vi "FaKI State Machine.vi"() -> ()   [LabVIEW 2021, in "FaKI State Machine.lvlib"]
doc: "The Producer-Consumer version of JKI State Machine.\n\nThis VI template must be instantiated by placing it on the block diagram of a new blank VI directly from the palettes. Do not use this template directly."
uses:
  FaKI State Machine.lvlib
panel:
  in  "Exit":bool
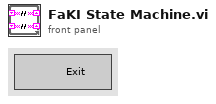
[diagram p1: front panel]
types:
  T1 = enum32{"Invalid", "Standard", "Closed", "Hidden", "Minimized", "Maximized"}
  T2 = enum32{"invalid app kind", "Development System", "Run Time System", "Student Edition", "Embedded LabVIEW", "Evaluation", "Custom"}
  T3 = cluster{"Core":cluster{"Current VI Reference":refnum<vi>, "Close Panel on Exit?":bool}, "Your Boolean data":bool, "Your string data":string}
  T4 = cluster{"Current VI Reference":refnum<vi>, "Close Panel on Exit?":bool}
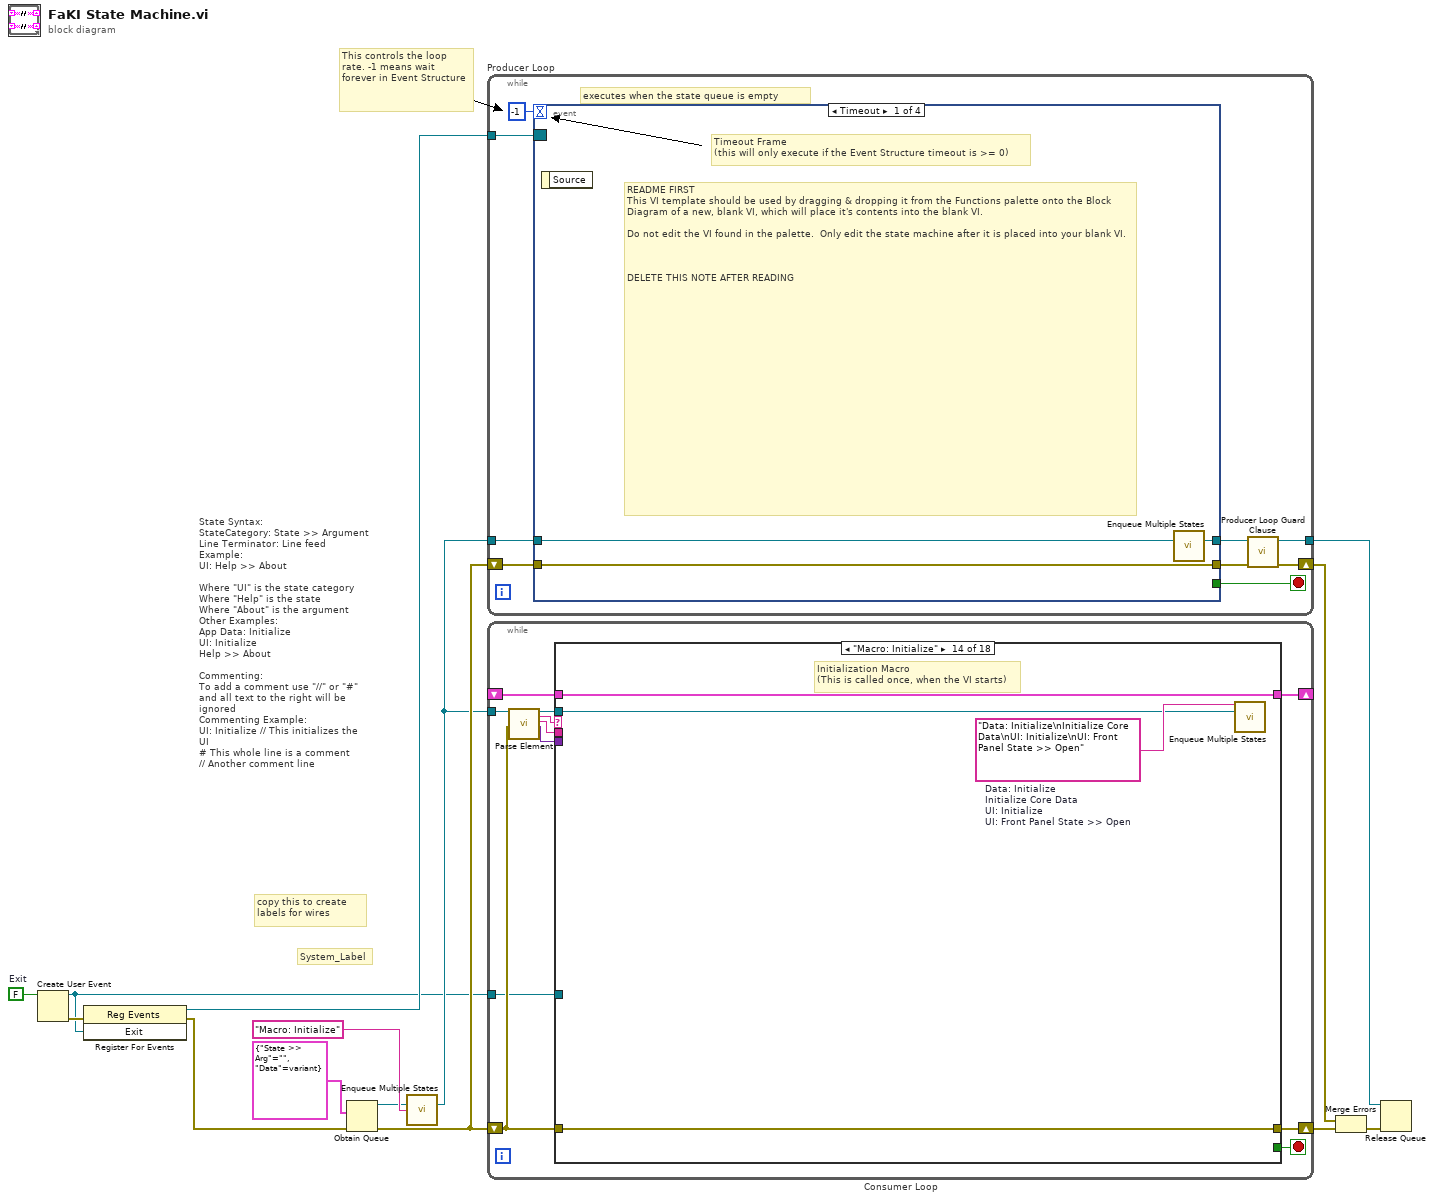
[diagram p0: block diagram]
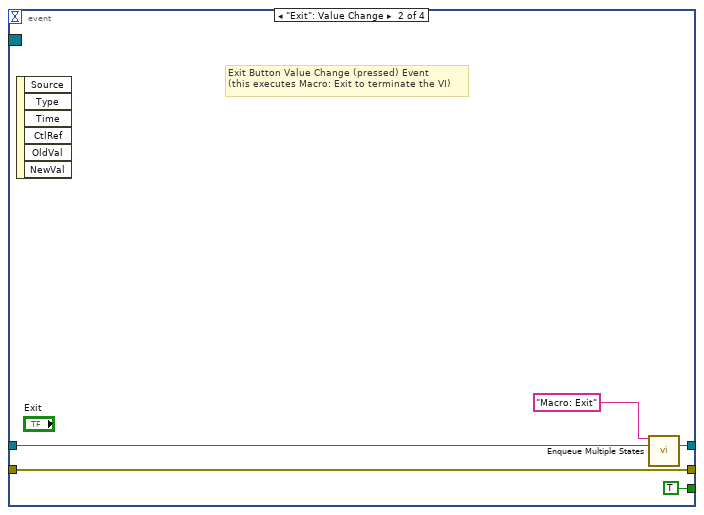
[diagram p2: hidden frame]
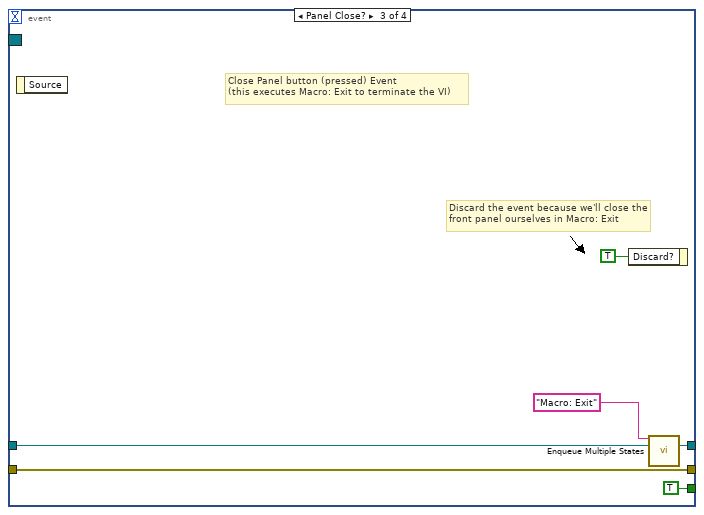
[diagram p3: hidden frame]
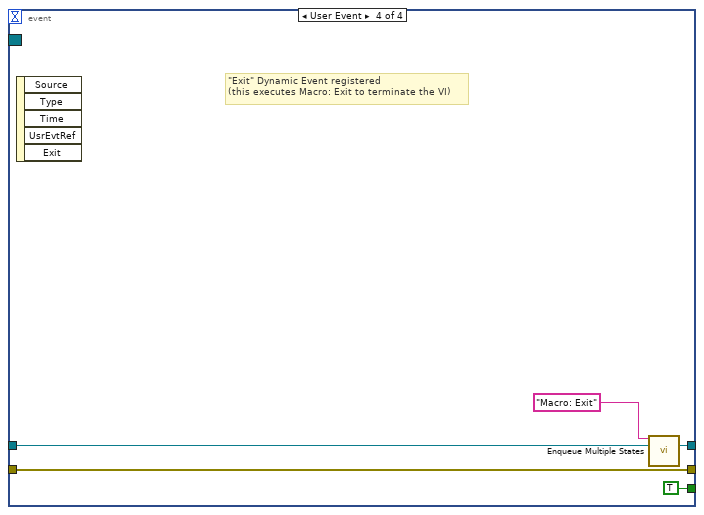
[diagram p4: hidden frame]
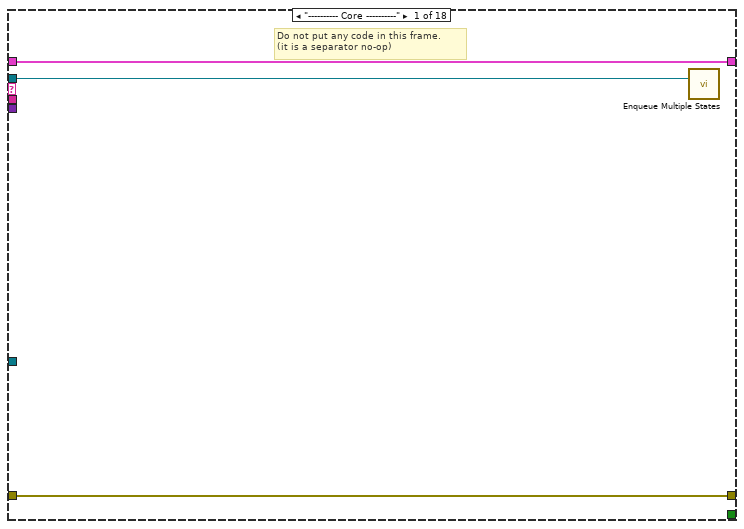
[diagram p5: hidden frame]
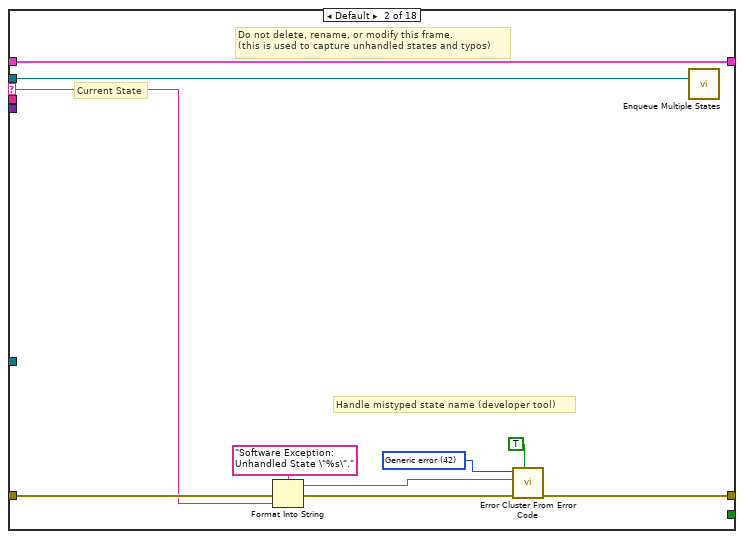
[diagram p6: hidden frame]
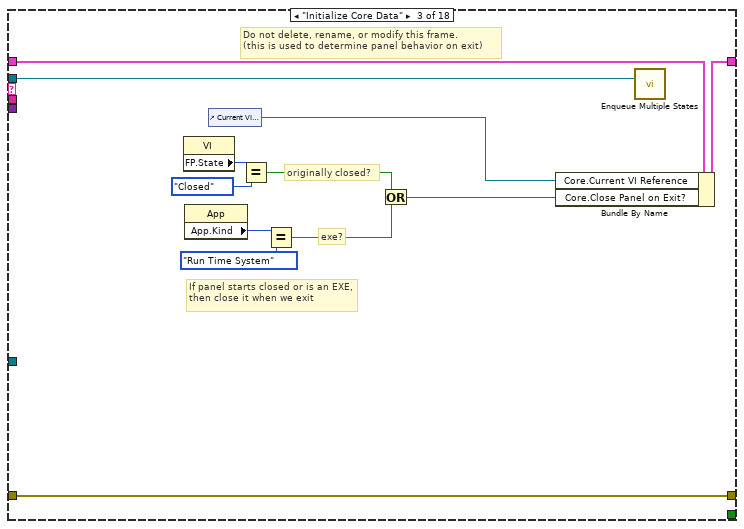
[diagram p7: hidden frame]
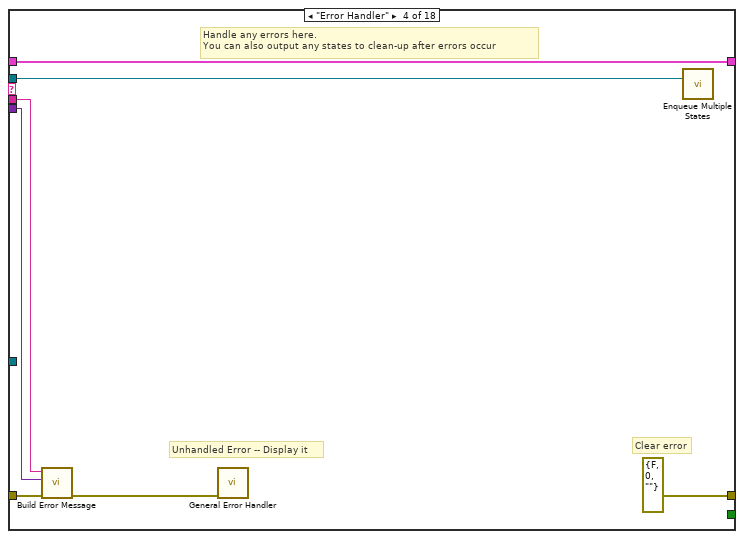
[diagram p8: hidden frame]
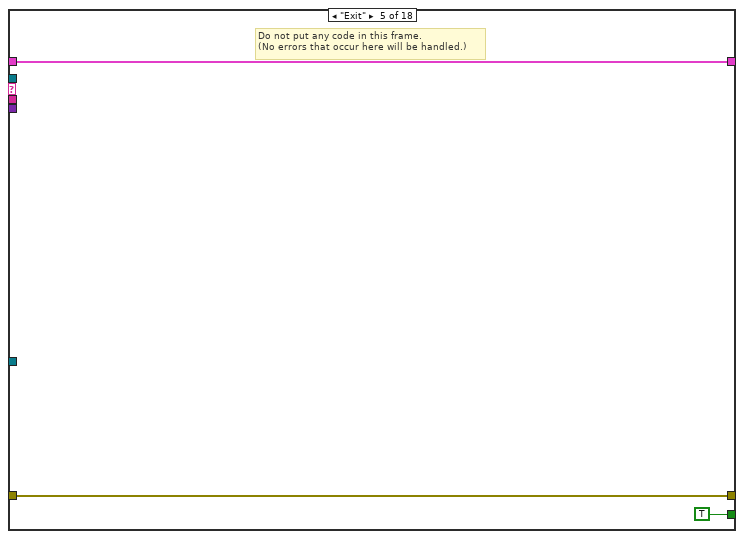
[diagram p9: hidden frame]
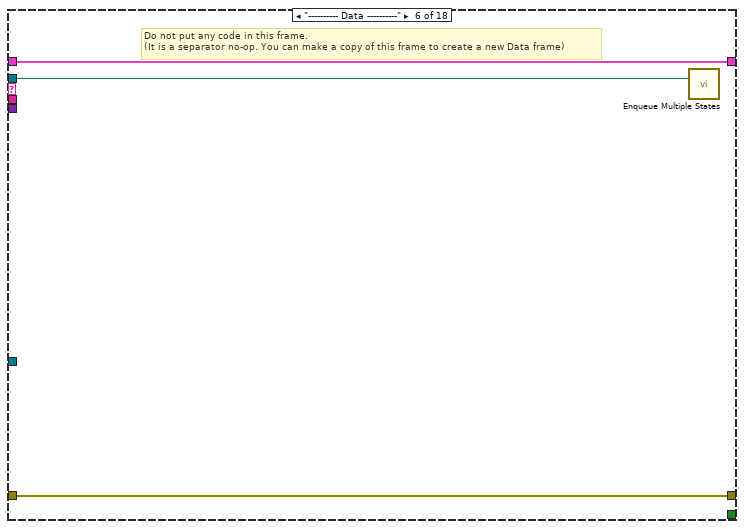
[diagram p10: hidden frame]
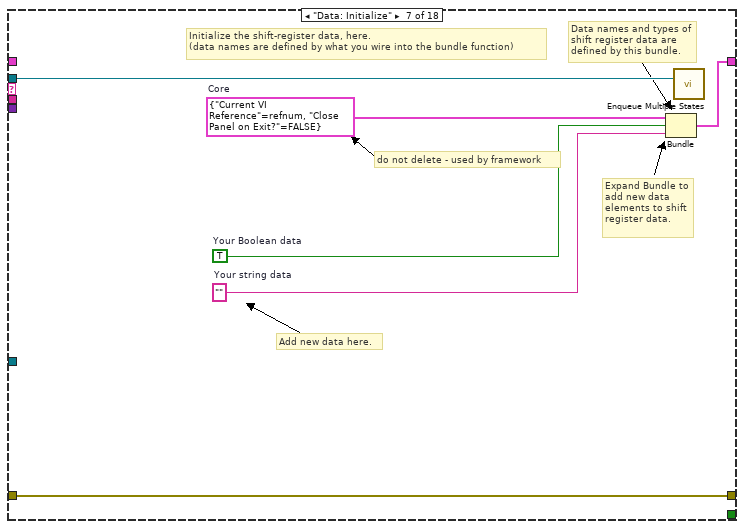
[diagram p11: hidden frame]
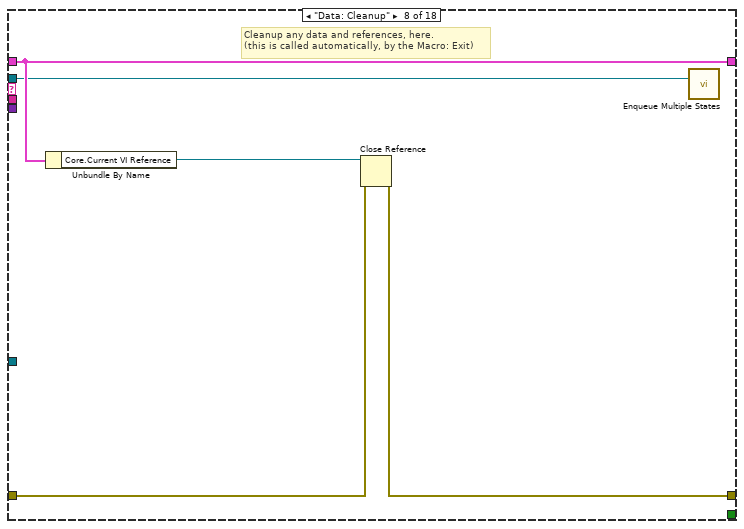
[diagram p12: hidden frame]
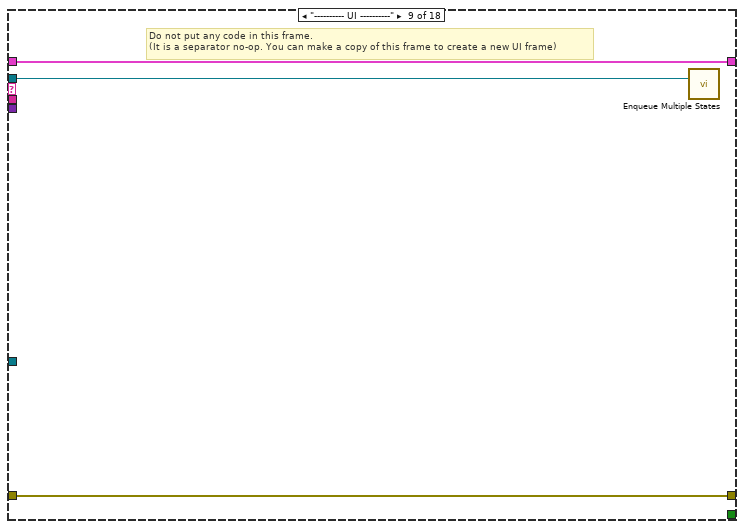
[diagram p13: hidden frame]
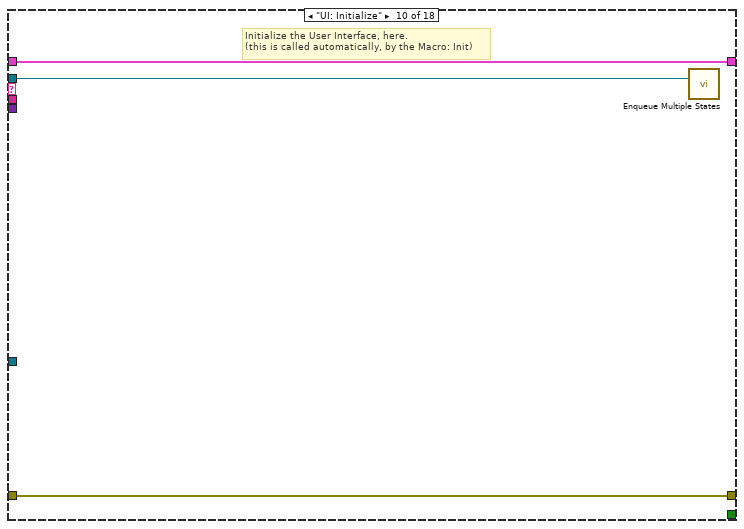
[diagram p14: hidden frame]
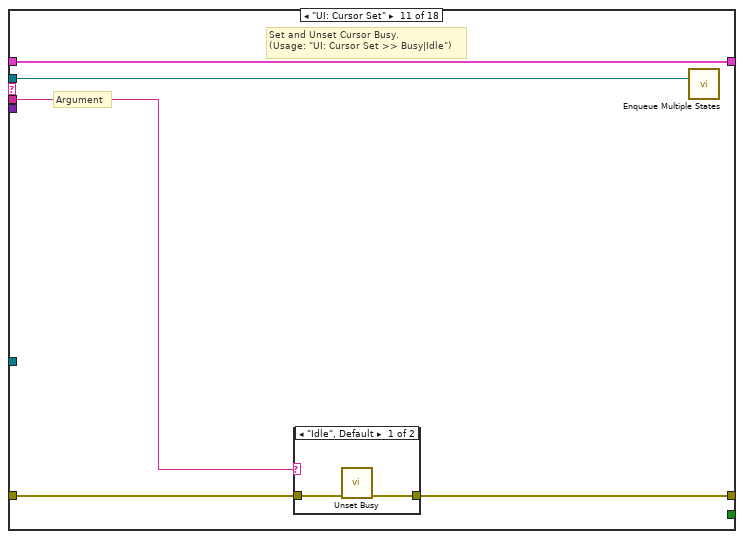
[diagram p15: hidden frame]
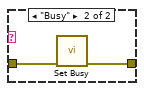
[diagram p16: hidden frame]
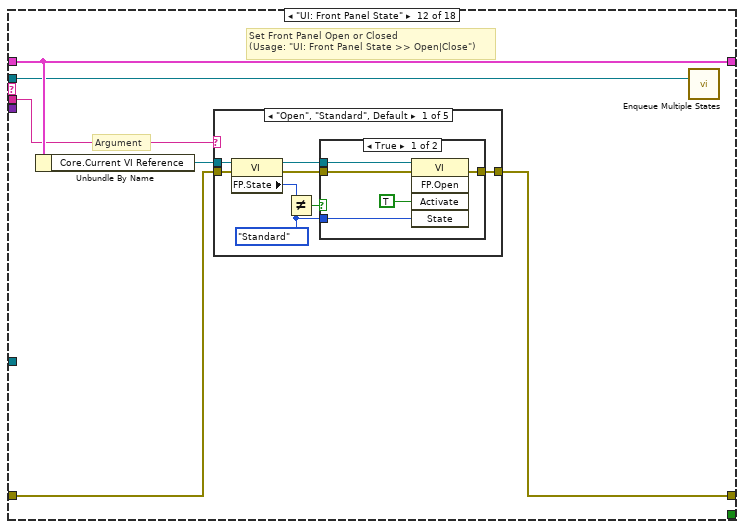
[diagram p17: hidden frame]
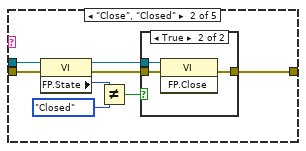
[diagram p19: hidden frame]
diagram:
  w4 = FALSE  # Exit
  # "This controls the loop rate. -1 means wait forever in Event Structure"
  # "State Syntax:\nStateCategory: State >> Argument\nLine Terminator: Line feed\nExample:\nUI: Help >> About\n\nWhere \"UI\" is the state category\nWhere \"Help\" is the state\nWhere \"About\" is the argument\nOther Examples:\nApp Data: Initialize\nUI: Initialize\nHelp >> About\n\nCommenting:\nTo add a comment use \"//\" or \"#\" and all text to the right will be ignored\nCommenting Example:\nUI: Initialize // This initializes the UI\n# This whole line is a comment\n// Another comment line"
  # "copy this to create labels for wires"
  # "System_Label"
  n1 = Create User Event(user event datatype=w4) -> (user event=w1:refnum<user-event>, error out=w5:errorcluster)  [unwired: 1 in]
  n2 = register-events(error in=w5, w1) -> (reference out=w2:refnum<event-registration>, error out=w3:errorcluster)  [unwired: 1 in]
  n3 = Obtain Queue(element data type=cluster{"State >> Arg":string, "Data":variant} {"State >> Arg"="", "Data"=variant}, error in (no error)=w3) -> (queue out=w11:refnum<queue>, error out=w14:errorcluster)  [unwired: 3 in, 1 out]
  n4 = call "Enqueue Multiple States.vi"("queue in"=w11, "State(s) at Back"="Macro: Initialize") -> ("queue out"=w10:refnum<queue>)  [unwired: 13 in]
  n5 = while "Producer Loop" {
    shift-right: [w18] -> w8
    shift-left: w14 -> [w23]
    tunnel: w2 -> [w15]
    tunnel: w10 -> [w21]
    tunnel: [w16] -> w6
    stop <- w20 stop-if-true
    # "executes when the state queue is empty"
    n6 = event shown="[0] Timeout" {
      selector: w15 -> [_ _ _ _]
      dyn-events: _ -> [_ _ _ _]
      timeout: -1 ("Timeout") -> [_ _ _ _]
      tunnel: [w24 w31 w37 w42] -> w19
      tunnel: w23 -> [w24 w31 w37 w42]
      tunnel: w21 -> [w25 w30 w34 w40]
      tunnel: [w26 w28 w33 w39] -> w17
      tunnel: [_ TRUE TRUE TRUE] -> w20
      event Timeout {
        # "README FIRST\nThis VI template should be used by dragging & dropping it from the Functions palette onto the Block Diagram of a new, blank VI, which will place it's contents into the blank VI.\n\nDo not edit the VI found in the palette.  Only edit the state machine after it is placed into your blank VI.\n\n\n\nDELETE THIS NOTE AFTER READING"
        # "Timeout Frame\n(this will only execute if the Event Structure timeout is >= 0)"
        n7 = event-data() -> ()  [unwired: 1 in, 1 out]
        n8 = call "Enqueue Multiple States.vi"("queue in"=w25) -> ("queue out"=w26:refnum<queue>)  [unwired: 14 in]
      }
      event "Exit": Value Change {
        # "Exit Button Value Change (pressed) Event\n(this executes Macro: Exit to terminate the VI)"
        n9 = event-data() -> ()  [unwired: 1 in, 6 out]
        n10 = call "Enqueue Multiple States.vi"("State(s) at Front"="Macro: Exit", "queue in"=w30) -> ("queue out"=w28:refnum<queue>)  [unwired: 13 in]
      }
      event Panel Close? {
        # "Discard the event because we'll close the front panel ourselves in Macro: Exit"
        # "Close Panel button (pressed) Event\n(this executes Macro: Exit to terminate the VI)"
        n11 = event-data() -> ()  [unwired: 1 in, 1 out]
        n12 = event-data("Discard?"=TRUE) -> ()  [unwired: 1 in, 1 out]
        n13 = call "Enqueue Multiple States.vi"("State(s) at Front"="Macro: Exit", "queue in"=w34) -> ("queue out"=w33:refnum<queue>)  [unwired: 13 in]
      }
      event User Event {
        # "\"Exit\" Dynamic Event registered\n(this executes Macro: Exit to terminate the VI)"
        n14 = event-data() -> ()  [unwired: 1 in, 5 out]
        n15 = call "Enqueue Multiple States.vi"("State(s) at Front"="Macro: Exit", "queue in"=w40) -> ("queue out"=w39:refnum<queue>)  [unwired: 13 in]
      }
    }
    n16 = call "Producer Loop Guard Clause.vi"("error in (no error)"=w19, "queue in"=w17) -> ("error out"=w18:errorcluster, "queue out"=w16:refnum<queue>)  [unwired: 8 in]
  }
  n17 = while "Consumer Loop" {
    shift-right: [w50] -> _
    shift-left: _ -> [w49]
    shift-right: [w53] -> w9
    shift-left: w14 -> [w52]
    tunnel: w10 -> [w48]
    tunnel: w1 -> [w43]
    stop <- w51 stop-if-true
    n18 = call "Parse Element.vi"("queue in"=w48, "error in (no error)"=w52) -> ("queue out"=w47:refnum<queue>, "State"=w46:string, "Arg"=w45:string, "Data"=w44:variant)  [unwired: 14 in]
    n19 = case shown="\"Macro: Initialize\"" w46 {
      selector: w46 -> [_ w58 _ _ _ _ _ _ _ _ _ _ _ _ _ _ _ _]
      tunnel: w47 -> [w54 w57 w67 w83 _ w89 w92 w98 w103 w106 w109 w118 w189 w192 w199 w205 w208 w211]
      tunnel: w45 -> [_ _ _ w79 _ _ _ _ _ _ w110 w119 _ _ _ _ _ _]
      tunnel: w49 -> [w55 w60 w73 w84 w87 w90 _ w99 w104 w107 w111 w121 w190 w194 w203 w206 w209 w212]
      tunnel: [w56 w65 w78 errorcluster {"status"=FALSE, "code"=0, "source"=""} ("error out") w88 w91 w97 w101 w105 w108 w112 w122 w191 w195 w204 w207 w210 w213] -> w53
      tunnel: w52 -> [w56 w64 w78 w82 w88 w91 w97 w102 w105 w108 w113 w123 w191 w195 w204 w207 w210 w213]
      tunnel: [_ _ _ _ TRUE _ _ _ _ _ _ _ _ _ _ _ _ _] -> w51
      tunnel: [w55 w60 w77 w84 w87 w90 w96 w99 w104 w107 w111 w121 w190 w194 w203 w206 w209 w212] -> w50
      tunnel: w44 -> [_ _ _ w80 _ _ _ _ _ _ _ _ _ _ _ _ _ _]
      tunnel: w43 -> [_ _ _ _ _ _ _ _ _ _ _ _ _ _ _ _ _ _]
      frame "---------- Core ----------" {
        # "Do not put any code in this frame.\n(it is a separator no-op)"
        n20 = call "Enqueue Multiple States.vi"("queue in"=w54) -> ()  [unwired: 14 in, 1 out]
      }
      frame Default {
        w62 = 42 items=["No error", "Argument error", "Memory is full", "Out of zone", "End of file", "File already open", "Generic file I/O error", "File not found", "File permission error", "Disk is full", "Duplicate path", "Too many files open", "System feature not enabled", "Resource file not found", "Cannot add resource", "Resource not found", "Image not found", "Image memory error", "Pen does not exist", "Config type invalid", "Config token not found", "Config parse error", "Config memory error", "Bad external code format", "Bad external code offset", "External code not present", "Null window", "Destroy window error", "Null menu", "Print aborted", "Bad print record", "Print driver error", "Windows error during printing", "Memory error during printing", "Print dialog error", "Generic print error", "Invalid device refnum", "Device not found", "Device parameter error", "Device unit error", "Cannot open device", "Device call aborted", "Generic error", "Cancelled by user", "Object ID too low", "Object ID too high", "Object not in heap", "Unknown heap", "Unknown object (invalid DefProc)", "Unknown object (DefProc not in table)", "Message out of range", "Invalid (null) method", "Unknown message", "Manager call not supported", "Bad address", "Network operation in progress", "Network operation timed out", "Connection is busy", "Network attribute not supported", "Network error", "Address in use", "System out of memory", "Connection aborted", "Connection refused", "Not connected", "Already connected", "Connection closed", "Initialization error (interapplication manager)", "Bad occurrence", "Wait on unbound occurrence handler", "Occurrence queue overflow", "Datalog type conflict", "Unused", "Unrecognized type (interapplication manager)", "Memory corrupt", "Failed to make temporary DLL", "Old CIN version", "Drag socket not found", "Failed to load drop-object", "Failed to register OLE object", "Failed to release OLE object", "Format specifier type mismatch", "Unknown format specifier", "Too few format specifiers", "Too many format specifiers", "Scan failed", "Newer CIN version", "Error converting to variant", "Runtime menu error", "Password tampered", "Variant attribute not found", "Incompatible variant data type", "Event data is not available", "Event Store is not present", "Occurrence is not found", "Event Queue is not created", "Event info is not available", "Refnum passed is NULL", "Error retrieving Class GUID", "Error retrieving CoClass GUID", "Error retrieving TypeLib GUID.", "Bad built application magic bytes.", "Specific driver is different from the specific driver associated with the Logical Name.", "There is no session opened to the class driver.", "Max Error", "MAX - Error with config objects", "MAX - Error loading configuration", "MAX - Group not supported"]
        # "Current State"
        # "Do not delete, rename, or modify this frame.\n(this is used to capture unhandled states and typos)"
        # "Handle mistyped state name (developer tool)"
        n21 = Format Into String(format string="Software Exception: Unhandled State \"%s\"." ("message"), error in=w64, w58) -> (resulting string=w61:string, error out=w66:errorcluster)  [unwired: 1 in]
        n22 = call <vilib>:"Error Cluster From Error Code.vi"("show call chain? (False)"=TRUE, "error in (no error)"=w66, "error message (\"\")"=w61, "error code (0)"=w62) -> ("error out"=w65:errorcluster)  [unwired: 5 in]
        n23 = call "Enqueue Multiple States.vi"("queue in"=w57) -> ()  [unwired: 14 in, 1 out]
      }
      frame "Initialize Core Data" {
        # "Do not delete, rename, or modify this frame.\n(this is used to determine panel behavior on exit)"
        # "originally closed?"
        # "exe?"
        # "If panel starts closed or is an EXE, then close it when we exit"
        n24 = property class="VI"() -> ("FP.State"=w70:T1)  [unwired: 2 in, 2 out]
        n25 = property class="App"() -> ("App.Kind"=w76:T2)  [unwired: 2 in, 2 out]
        n26 = control-ref of="Current VI Reference"() -> (w71:refnum<vi>)
        n27 = Equal?(x=w70, y=T1."Closed" ("Front Panel Window:State")) -> (x = y?=w68:bool)
        n28 = Equal?(x=w76, y=T2."Run Time System" ("Application:Kind")) -> (x = y?=w74:bool)
        n29 = Or(x=w68, y=w74) -> (x .or. y?=w72:bool)
        n30 = Bundle By Name(cluster=w73, "Core.Current VI Reference"=w71, "Core.Close Panel on Exit?"=w72) -> (w77:T3)
        n31 = call "Enqueue Multiple States.vi"("queue in"=w67) -> ()  [unwired: 14 in, 1 out]
      }
      frame "Error Handler" {
        # "Unhandled Error -- Display it"
        # "Handle any errors here.\nYou can also output any states to clean-up after errors occur"
        # "Clear error"
        n32 = call "Build Error Message.vi"("error in (no error)"=w82, "Data"=w80, "Arg"=w79) -> ("error out"=w81:errorcluster)  [unwired: 8 in]
        n33 = call <vilib>:"General Error Handler.vi"("error in (no error)"=w81) -> ()  [unwired: 10 in, 5 out]
        n34 = call "Enqueue Multiple States.vi"("queue in"=w83) -> ()  [unwired: 14 in, 1 out]
      }
      frame "Exit" {
        # "Do not put any code in this frame.\n(No errors that occur here will be handled.)"
      }
      frame "---------- Data ----------" {
        # "Do not put any code in this frame.\n(It is a separator no-op. You can make a copy of this frame to create a new Data frame)"
        n35 = call "Enqueue Multiple States.vi"("queue in"=w89) -> ()  [unwired: 14 in, 1 out]
      }
      frame "Data: Initialize" {
        w93 = T4 {"Current VI Reference"=refnum, "Close Panel on Exit?"=FALSE}  # Core
        w95 = TRUE  # Your Boolean data
        w94 = ""  # Your string data
        # "do not delete - used by framework"
        # "Expand Bundle to add new data elements to shift register data."
        # "Add new data here."
        # "Data names and types of shift register data are defined by this bundle."
        # "Initialize the shift-register data, here.\n(data names are defined by what you wire into the bundle function)"
        n36 = Bundle("Core"=w93, "Your Boolean data"=w95, "Your string data"=w94) -> (w96:T3)  [unwired: 1 in]
        n37 = call "Enqueue Multiple States.vi"("queue in"=w92) -> ()  [unwired: 14 in, 1 out]
      }
      frame "Data: Cleanup" {
        # "Cleanup any data and references, here.\n(this is called automatically, by the Macro: Exit)"
        n38 = Unbundle By Name(w99) -> ("Core.Current VI Reference"=w100:refnum<vi>)
        n39 = Close Reference(reference=w100, error in (no error)=w102) -> (error out=w101:errorcluster)
        n40 = call "Enqueue Multiple States.vi"("queue in"=w98) -> ()  [unwired: 14 in, 1 out]
      }
      frame "---------- UI ----------" {
        # "Do not put any code in this frame.\n(It is a separator no-op. You can make a copy of this frame to create a new UI frame)"
        n41 = call "Enqueue Multiple States.vi"("queue in"=w103) -> ()  [unwired: 14 in, 1 out]
      }
      frame "UI: Initialize" {
        # "Initialize the User Interface, here.\n(this is called automatically, by the Macro: Init)"
        n42 = call "Enqueue Multiple States.vi"("queue in"=w106) -> ()  [unwired: 14 in, 1 out]
      }
      frame "UI: Cursor Set" {
        # "Argument"
        # "Set and Unset Cursor Busy.\n(Usage: \"UI: Cursor Set >> Busy|Idle\")"
        n43 = case shown="\"Idle\", Default" w110 {
          tunnel: w113 -> [w115 w117]
          tunnel: [w114 w116] -> w112
          frame "Idle", Default {
            n44 = call <vilib>:"Unset Busy.vi"("error in (no error)"=w115) -> ("error out"=w114:errorcluster)  [unwired: 10 in]
          }
          frame "Busy" {
            n45 = call <vilib>:"Set Busy.vi"("error in (no error)"=w117) -> ("error out"=w116:errorcluster)  [unwired: 9 in, 1 out]
          }
        }
        n46 = call "Enqueue Multiple States.vi"("queue in"=w109) -> ()  [unwired: 14 in, 1 out]
      }
      frame "UI: Front Panel State" {
        # "Argument"
        # "Set Front Panel Open or Closed\n(Usage: \"UI: Front Panel State >> Open|Close\")"
        n47 = Unbundle By Name(w121) -> ("Core.Current VI Reference"=w120:refnum<vi>)
        n48 = case shown="\"Open\", \"Standard\", Default" w119 {
          tunnel: w123 -> [w130 w144 w156 w169 w182]
          tunnel: [w131 w145 w157 w170 w183] -> w122
          tunnel: w120 -> [w128 w142 w154 w167 w180]
          frame "Open", "Standard", Default {
            w124 = T1."Standard" ("State")
            n49 = property class="VI"(reference=w128, error in=w130) -> (reference out=w127:refnum<vi>, error out=w129:errorcluster, "FP.State"=w126:T1)
            n50 = Not Equal?(x=w126, y=w124) -> (x != y?=w125:bool)
            n51 = case shown="True" w125 {
              tunnel: [w136 w137] -> w131
              tunnel: w129 -> [w135 w137]
              tunnel: w127 -> [w133 _]
              tunnel: w124 -> [w132 _]
              frame True {
                n52 = invoke class="VI" method="FP.Open"(reference=w133, error in=w135, "Activate"=TRUE, "State"=w132) -> (error out=w136:errorcluster)  [unwired: 1 in, 4 out]
              }
              frame False {
              }
            }
          }
          frame "Close", "Closed" {
            n53 = property class="VI"(reference=w142, error in=w144) -> (reference out=w141:refnum<vi>, error out=w143:errorcluster, "FP.State"=w139:T1)
            n54 = Not Equal?(x=w139, y=T1."Closed" ("Front Panel Window:State")) -> (x != y?=w138:bool)
            n55 = case shown="True" w138 {
              tunnel: [w146 w149] -> w145
              tunnel: w143 -> [w146 w148]
              tunnel: w141 -> [_ w147]
              frame False {
              }
              frame True {
                n56 = invoke class="VI" method="FP.Close"(reference=w147, error in=w148) -> (error out=w149:errorcluster)  [unwired: 1 in, 2 out]
              }
            }
          }
          frame "Hidden", "Hide" {
            w150 = T1."Hidden" ("State")
            n57 = property class="VI"(reference=w154, error in=w156) -> (reference out=w153:refnum<vi>, error out=w155:errorcluster, "FP.State"=w152:T1)
            n58 = Not Equal?(x=w152, y=w150) -> (x != y?=w151:bool)
            n59 = case shown="True" w151 {
              tunnel: [w161 w162] -> w157
              tunnel: w155 -> [w160 w162]
              tunnel: w153 -> [w159 _]
              tunnel: w150 -> [w158 _]
              frame True {
                n60 = invoke class="VI" method="FP.Open"(reference=w159, error in=w160, "State"=w158) -> (error out=w161:errorcluster)  [unwired: 2 in, 4 out]
              }
              frame False {
              }
            }
          }
          frame "Minimize", "Minimized" {
            w163 = T1."Minimized" ("State")
            n61 = property class="VI"(reference=w167, error in=w169) -> (reference out=w166:refnum<vi>, error out=w168:errorcluster, "FP.State"=w165:T1)
            n62 = Not Equal?(x=w165, y=w163) -> (x != y?=w164:bool)
            n63 = case shown="True" w164 {
              tunnel: [w174 w175] -> w170
              tunnel: w168 -> [w173 w175]
              tunnel: w166 -> [w172 _]
              tunnel: w163 -> [w171 _]
              frame True {
                n64 = invoke class="VI" method="FP.Open"(reference=w172, error in=w173, "State"=w171) -> (error out=w174:errorcluster)  [unwired: 2 in, 4 out]
              }
              frame False {
              }
            }
          }
          frame "Maximize", "Maximized" {
            w176 = T1."Maximized" ("State")
            n65 = property class="VI"(reference=w180, error in=w182) -> (reference out=w179:refnum<vi>, error out=w181:errorcluster, "FP.State"=w178:T1)
            n66 = Not Equal?(x=w178, y=w176) -> (x != y?=w177:bool)
            n67 = case shown="True" w177 {
              tunnel: [w187 w188] -> w183
              tunnel: w181 -> [w186 w188]
              tunnel: w179 -> [w185 _]
              tunnel: w176 -> [w184 _]
              frame True {
                n68 = invoke class="VI" method="FP.Open"(reference=w185, error in=w186, "State"=w184) -> (error out=w187:errorcluster)  [unwired: 2 in, 4 out]
              }
              frame False {
              }
            }
          }
        }
        n69 = call "Enqueue Multiple States.vi"("queue in"=w118) -> ()  [unwired: 14 in, 1 out]
      }
      frame "---------- Macro ----------" {
        # "Do not put any code in this frame.\n(It is a separator no-op. You can make a copy of this frame to create a new Macro frame)"
        n70 = call "Enqueue Multiple States.vi"("queue in"=w189) -> ()  [unwired: 14 in, 1 out]
      }
      frame "Macro: Initialize" {
        w193 = "Data: Initialize\nInitialize Core Data\nUI: Initialize\nUI: Front Panel State >> Open"  # Data: Initialize Initialize Core Data UI: Initialize UI: Front Panel State >> Open
        # "Initialization Macro\n(This is called once, when the VI starts)"
        n71 = call "Enqueue Multiple States.vi"("State(s) at Front"=w193, "queue in"=w192) -> ()  [unwired: 13 in, 1 out]
      }
      frame "Macro: Exit" {
        # "Exit Macro\n(This is called once, when the VI exits)"
        n72 = Unbundle By Name(w203) -> ("Core.Close Panel on Exit?"=w202:bool)
        n73 = Select(t="UI: Front Panel State >> Close\n", s=w202, f="") -> (s? t:f=w198:string)
        n74 = Concatenate Strings(w198, "Data: Cleanup\nExit") -> (w196:string)
        n75 = call "Enqueue Multiple States.vi"("State(s) at Front"=w196, "queue in"=w199) -> ()  [unwired: 13 in, 1 out]
      }
      frame "---------- New Category ----------" {
        # "Template Separator\n(You can make a copy of, or modify, this frame)"
        n76 = call "Enqueue Multiple States.vi"("queue in"=w205) -> ()  [unwired: 14 in, 1 out]
      }
      frame "New Category: 1" {
        # "Your code here.\n(You can make a copy of, or modify, this frame)"
        n77 = call "Enqueue Multiple States.vi"("queue in"=w208) -> ()  [unwired: 14 in, 1 out]
      }
      frame "New Category: 2" {
        # "Your code here.\n(You can make a copy of, or modify, this frame)"
        n78 = call "Enqueue Multiple States.vi"("queue in"=w211) -> ()  [unwired: 14 in, 1 out]
      }
    }
  }
  n79 = Merge Errors(w8, w9) -> (w7:errorcluster)
  n80 = Release Queue(queue=w6, error in (no error)=w7) -> ()  [unwired: 1 in, 3 out]
